vi "USBData_read.vi"(6 "error in (no error)":errorcluster, 9 "USBData in":refnum<class "USBData.lvclass">) -> (0 "error out":errorcluster, 1 "FileRefs":T1, 2 "Data":T2, 3 "USBData out":refnum<class "USBData.lvclass">, 4 "DAQsettings":T3, 5 "Basic":T4)   [LabVIEW 2017, in "USBData.lvclass"]
uses:
  USBData.lvclass
  USBData.lvclass/USBData.ctl
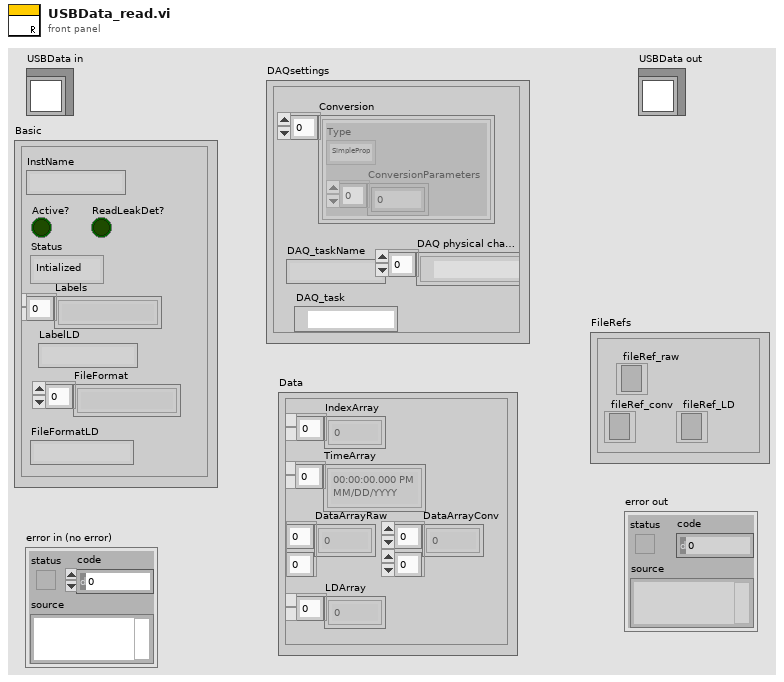
[diagram p1: front panel]
types:
  T1 = cluster{"fileRef_raw":refnum<file>, "fileRef_conv":refnum<file>, "fileRef_LD":refnum<file>}
  T2 = cluster{"IndexArray":i64[], "TimeArray":timestamp[], "DataArrayRaw":dbl[][], "DataArrayConv":dbl[][], "LDArray":dbl[]}
  T3 = cluster{"Conversion":cluster{"Type":enum16{"SimpleProp", "CC-10_COMBINED", "CC-10_LOG", "LeakDet_EXP", "LeakDet_Mantissa", "Baratron"}, "ConversionParameters":dbl[]}[], "DAQ_taskName":string, "DAQ_task":refnum<k21>, "DAQ physical channels":tag[]}
  T4 = cluster{"InstName":string, "Active?":bool, "Status":enum16{"Intialized", "Waiting", "Measuring", "Terminated"}, "Labels":string[], "LabelLD":string, "FileFormat":string[], "FileFormatLD":string, "ReadLeakDet?":bool}
  T5 = enum16{"Intialized", "Waiting", "Measuring", "Terminated"}
  T6 = cluster{"Type":enum16{"SimpleProp", "CC-10_COMBINED", "CC-10_LOG", "LeakDet_EXP", "LeakDet_Mantissa", "Baratron"}, "ConversionParameters":dbl[]}[]
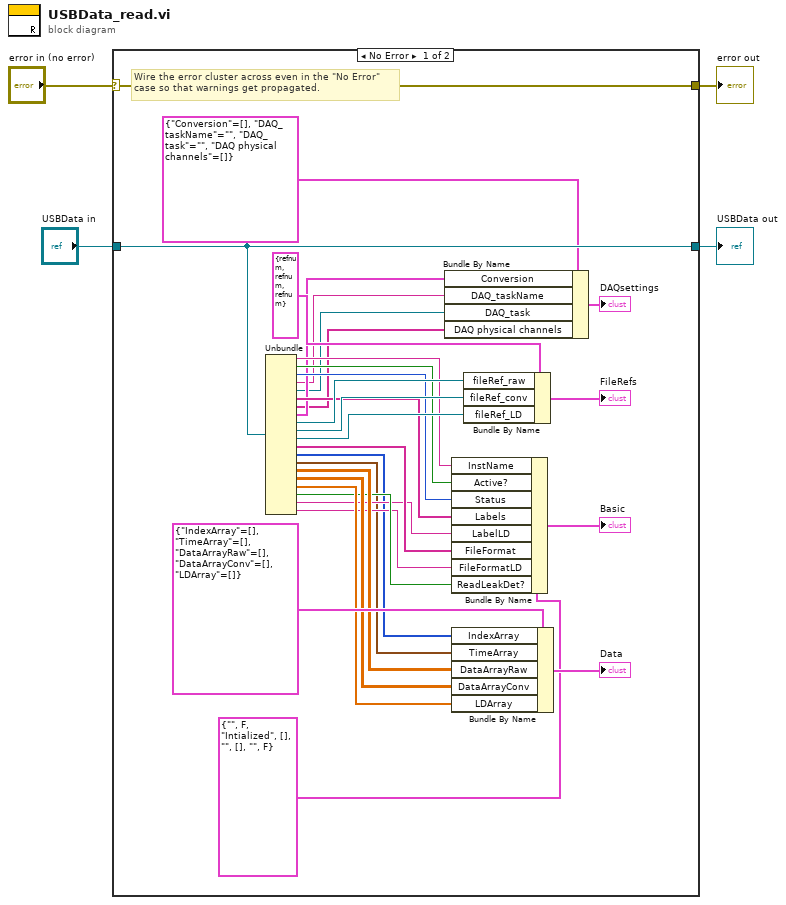
[diagram p0: block diagram]
diagram:
  n1 = case shown="No Error" "error in (no error)" {
    selector: "error in (no error)" -> [w34 w36]
    tunnel: [w34 w36] -> w3
    tunnel: [w33 w35] -> w1
    tunnel: "USBData in" -> [w33 w35]
    frame No Error {
      # "Wire the error cluster across even in the \"No Error\"\ncase so that warnings get propagated."
      n2 = Unbundle(w33) -> (w20:string, w19:bool, w18:T5, w9:string, w8:refnum<k21>, w17:string[], w7:tag[], w10:T6, w30:refnum<file>, w29:refnum<file>, w28:refnum<file>, w14:string[], w6:i64[], w5:timestamp[], w25:dbl[][], w24:dbl[][], w23:dbl[], w16:bool, w13:string, w15:string)
      n3 = Bundle By Name(cluster=T3 {"Conversion"=[], "DAQ_taskName"="", "DAQ_task"="", "DAQ physical channels"=[]} ("DAQsettings 2"), "Conversion"=w10, "DAQ_taskName"=w9, "DAQ_task"=w8, "DAQ physical channels"=w7) -> (→"DAQsettings":T3)
      n4 = Bundle By Name(cluster=T4 {"InstName"="", "Active?"=FALSE, "Status"=enum."Intialized", "Labels"=[], "LabelLD"="", "FileFormat"=[], "FileFormatLD"="", "ReadLeakDet?"=FALSE} ("Basic 2"), "InstName"=w20, "Active?"=w19, "Status"=w18, "Labels"=w17, "LabelLD"=w13, "FileFormat"=w14, "FileFormatLD"=w15, "ReadLeakDet?"=w16) -> (→"Basic":T4)
      n5 = Bundle By Name(cluster=T2 {"IndexArray"=[], "TimeArray"=[], "DataArrayRaw"=[], "DataArrayConv"=[], "LDArray"=[]} ("Data 2"), "IndexArray"=w6, "TimeArray"=w5, "DataArrayRaw"=w25, "DataArrayConv"=w24, "LDArray"=w23) -> (→"Data":T2)
      n6 = Bundle By Name(cluster=T1 {"fileRef_raw"=refnum, "fileRef_conv"=refnum, "fileRef_LD"=refnum} ("FileRefs 2"), "fileRef_raw"=w30, "fileRef_conv"=w29, "fileRef_LD"=w28) -> (→"FileRefs":T1)
    }
    frame Error {
    }
  }
  "error out" <- w3
  "USBData out" <- w1
